vi "Obtain Reentrant VI Queue.vi"(10 "error in (no error)":errorcluster, 11 "Name":string) -> (2 "error out":errorcluster, 3 "queue out":refnum<queue>)   [LabVIEW 2018, in "Dynamic Reentrant.lvlib"]
uses:
  <userlib>/Dynamic Reentrant/Dynamic Reentrant.lvlib
  <userlib>/Dynamic Reentrant/Type Defs/Message.ctl
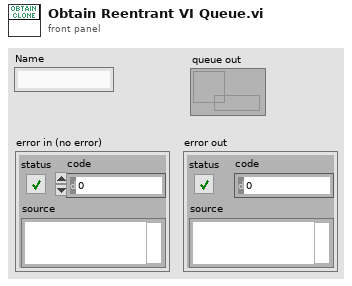
[diagram p1: front panel]
types:
  T1 = typedef "Dynamic Reentrant.lvlib/Message.ctl" = cluster{"Source":string, "Destination":string, "Time Stamp":timestamp, "Command":string, "Data":variant}
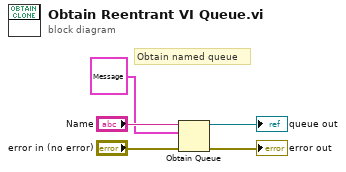
[diagram p0: block diagram]
diagram:
  # "Obtain named queue"
  n1 = Obtain Queue(name (unnamed)="Name", element data type=T1 {"Source"="", "Destination"="", "Time Stamp"=timestamp(0 s since 1904-01-01), "Command"="", "Data"=variant(string "")} ("Message"), error in (no error)="error in (no error)") -> (queue out=→"queue out":refnum<queue>, error out=→"error out":errorcluster)  [unwired: 2 in, 1 out]
